vi "Trajectory_Controller.vi"(0 "Error In":errorcluster, 1 "reset":dbl, 2 "Interpolation activator":bool, 3 "Abort Trajectory":bool, 4 "Controller Data In":refnum<data-value>, 5 "Configuration":T1={"Accelerometer Bias"={"X (m/s)"=0.0, "Y (m/s)"=0.0, "Z (m/s)"=0.0}, "Gyroscope Bias"={"X (m/s)"=0.0, "Y (m/s)"=0.0, "Z (m/s)"=0.0}, "Steering Motor Gear Ratio"=611.0, "Steering Pully Gear Ratio"=1.0, "Steering Encoder CPR"=500.0, "Steering Motor Max RPM"=4000.0, "Wheelbase (m)"=1.12, "Fork Angle (rad)"=1.3, "Balancing Controller"={"Kp (/s)"=1.0, "Kd (1)"=1.0}, "Max Allowed Steering Angle (rad)"=0.7, "Task Periods"={"Emergency Stop (us)"=10000, "IMU (us)"=10000, "Steering Motor Encoder (us)"=10000, "State Estimator (us)"=10000, "Balancing Controller (us)"=10000, "GNSS (us)"=10000, "Logging (us)"=50000, "Drive Motor (us)"=100000, "Visualization (us)"=50000}, "Drive Motor Gear Ratio"=0.7, "lr"=0.0, "lf"=0.0, "lambda"=0.0, "k1"=0.0, "k2"=0.0, "e1_max"=0.0, "Ad_tmin"=0.0, "Bd_tmin"=0.0, "C_tmin"=0.0, "D_tmin"=0.0, "Wheel radius"=0.311, "Ad_tmax"=0.95971, "Bd_tmax"=0.01, "C_tmax"=2.20588, "D_tmax"=0.0, "Vmin"=2.20588, "Vmax"=0.0}, 7 "State Estimate In":refnum<data-value>, 8 "Constant V matrixmat":dbl, 9 "Reset and Init trajectory":bool, 11 "RefTraj in":refnum<data-value>, 12 "Trajectory In":refnum<data-value>, 13 "Measurement In":refnum<data-value>) -> (6 "Error out":errorcluster, 10 "Trajectory Out":refnum<data-value>, 14 "E1 limit":bool, 15 "E2 limit":bool)   [LabVIEW 2021]
uses:
  State Estimator/State Estimate.ctl
  Trajectory_Control.ctl
  Configuration/Configuration.ctl
  State Estimator/Measurements.ctl
  IMU/IMU Data.ctl
  Steering Motor Encoder/Steering Motor Encoder Data.ctl
  GNSS/GNSS Data.ctl
  Logging/Controller Data.ctl
  Drive Motor/Drive Motor Data.ctl
  Steering Motor/Steering Motor Data.ctl
panel:
  out "Numeric":dbl
  out "Controller Data Out":refnum<data-value>
  out "lat_con":dbl
  out "head con":dbl
  out "delta":dbl
  out "State Estimate Out":refnum<data-value>
  out "RefTraj out":refnum<data-value>
  out "Measurement Out":refnum<data-value>
  out "size(s)":i32[](array[numeric])
  out "error2":dbl
  out "error1":dbl
  out "Rollref":dbl
  out "Closestpoint":dbl
  in  "path in":path=path "libtrajectory_controller.so"
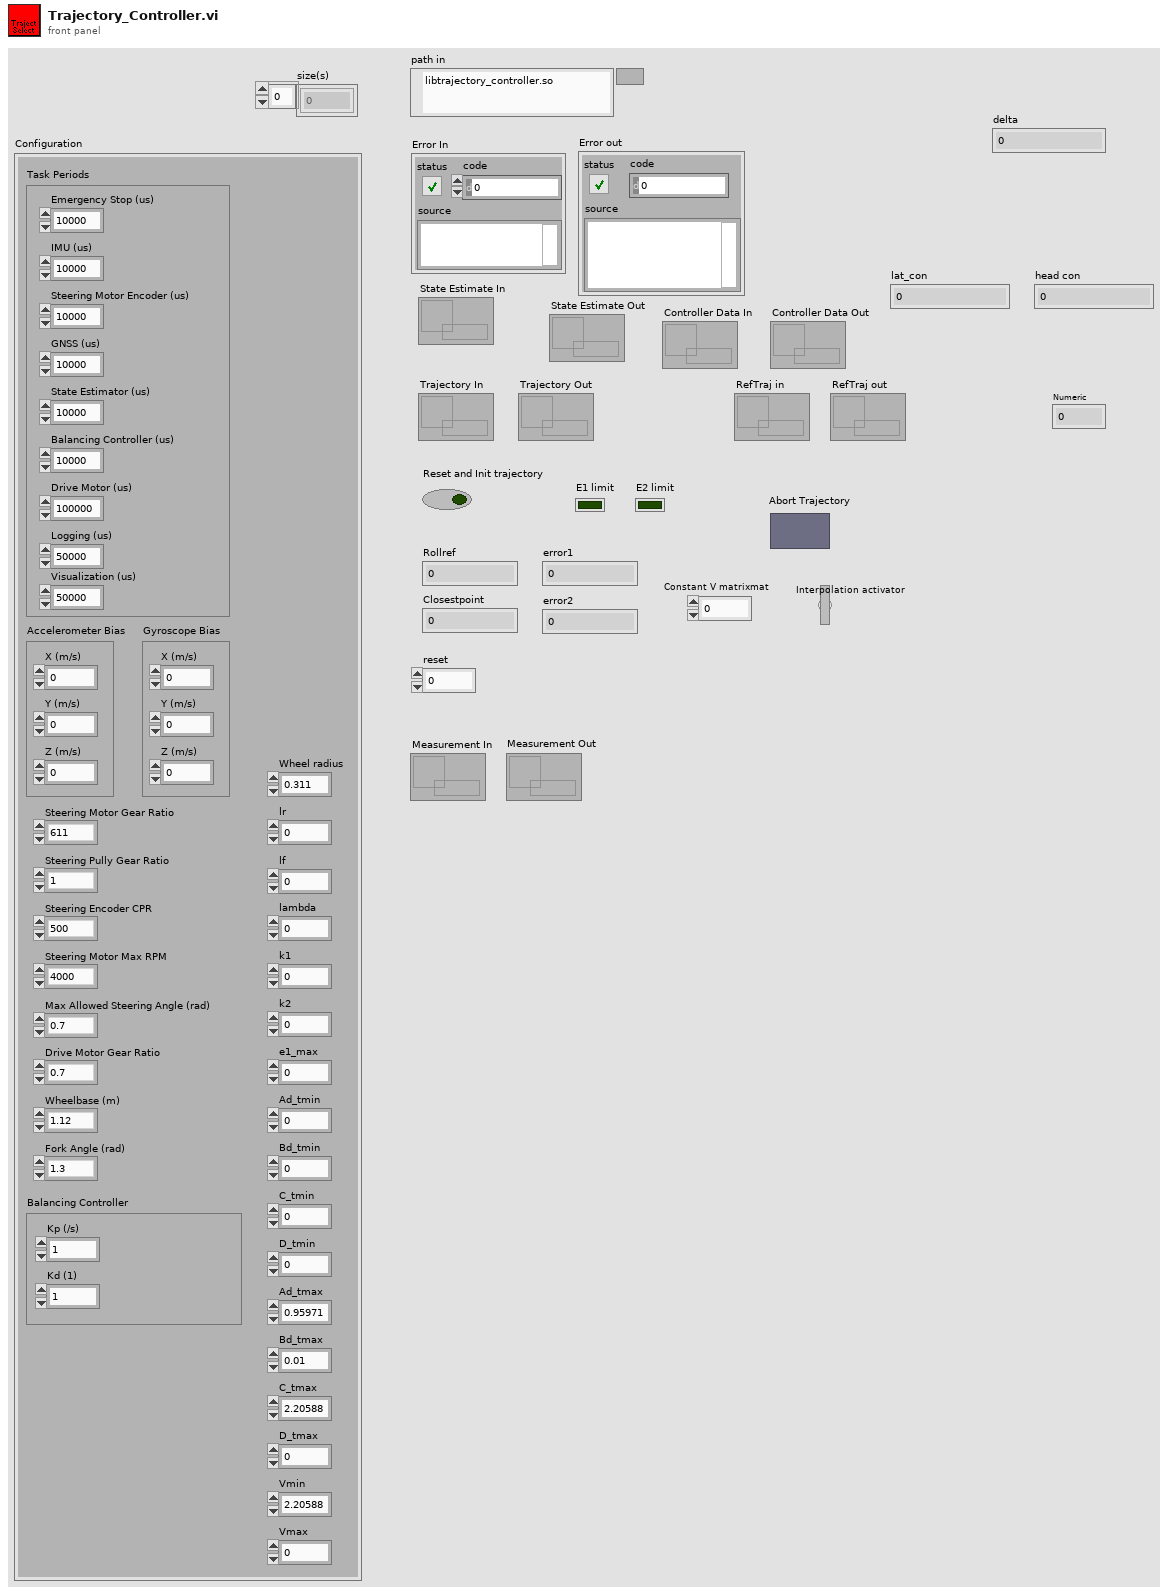
[diagram p1: front panel]
types:
  T1 = typedef "Configuration.ctl" = cluster{"Accelerometer Bias":cluster{"X (m/s)":dbl, "Y (m/s)":dbl, "Z (m/s)":dbl}, "Gyroscope Bias":cluster{"X (m/s)":dbl, "Y (m/s)":dbl, "Z (m/s)":dbl}, "Steering Motor Gear Ratio":dbl, "Steering Pully Gear Ratio":dbl, "Steering Encoder CPR":dbl, "Steering Motor Max RPM":dbl, "Wheelbase (m)":dbl, "Fork Angle (rad)":dbl, "Balancing Controller":cluster{"Kp (/s)":dbl, "Kd (1)":dbl}, "Max Allowed Steering Angle (rad)":dbl, "Task Periods":cluster{"Emergency Stop (us)":i64, "IMU (us)":i64, "Steering Motor Encoder (us)":i64, "State Estimator (us)":i64, "Balancing Controller (us)":i64, "GNSS (us)":i64, "Logging (us)":i64, "Drive Motor (us)":i64, "Visualization (us)":i64}, "Drive Motor Gear Ratio":dbl, "lr":dbl, "lf":dbl, "lambda":dbl, "k1":dbl, "k2":dbl, "e1_max":dbl, "Ad_tmin":dbl, "Bd_tmin":dbl, "C_tmin":dbl, "D_tmin":dbl, "Wheel radius":dbl, "Ad_tmax":dbl, "Bd_tmax":dbl, "C_tmax":dbl, "D_tmax":dbl, "Vmin":dbl, "Vmax":dbl}
  T2 = typedef "Trajectory_Control.ctl" = cluster{"Rollref":dbl, "Closestpoint":dbl, "Error1":dbl, "Error2":dbl, "Dpsiref_cont":dbl, "Lateral_cont":dbl, "Heading_cont":dbl, "Reset_traj":dbl, "Iteration":dbl, "E1 limit":u32, "E2 limit":u32, "Vref":dbl}
  T3 = typedef "Measurements.ctl" = cluster{"IMU Data":T4, "Steering Motor Encoder Data":T5, "GNSS Data":T6}
  T4 = typedef "IMU Data.ctl" = cluster{"Gyroscope":cluster{"X (rad/s)":dbl, "Y (rad/s)":dbl, "Z (rad/s)":dbl}, "Accelerometer":cluster{"X (m/s^2)":dbl, "Y (m/s^2)":dbl, "Z (m/s^2)":dbl}, "Flag IMU":dbl}
  T5 = typedef "Steering Motor Encoder Data.ctl" = cluster{"Encoder Position (counts)":i32, "Steering Angle (rad)":dbl, "Steering Encoder Iteration":dbl}
  T6 = typedef "GNSS Data.ctl" = cluster{"Latitude (rad)":dbl, "Longitude (rad)":dbl, "Altitude (m)":dbl, "Speed (m/s)":dbl, "Heading (rad)":dbl, "Fix Quality":i32, "Number of Satellites":i32, "Latitude (deg)":dbl, "Longitude (deg)":dbl, "Flag GNSS":dbl}
  T7 = typedef "Controller Data.ctl" = cluster{"Drive Motor Data":T8, "Steering Motor Data":T9}
  T8 = typedef "Drive Motor Data.ctl" = cluster{"Angular Speed (rad/s)":dbl, "Input Current (A)":dbl, "Motor Current (A)":dbl, "MOSFET Temperature (deg C)":dbl, "Reference Speed (rad/s)":dbl, "PI Current (A)":dbl, "Ki":dbl, "Kp":dbl}
  T9 = typedef "Steering Motor Data.ctl" = cluster{"PWM":dbl, "Steering Angle Rate (rad/s)":dbl, "input balancing":dbl}
  T10 = typedef "State Estimate.ctl" = cluster{"X (m)":dbl, "Y (m)":dbl, "Psi (rad)":dbl, "Roll (rad)":dbl, "Roll Rate (rad/s)":dbl, "delta":dbl, "velocity":dbl, "Iterations":dbl}
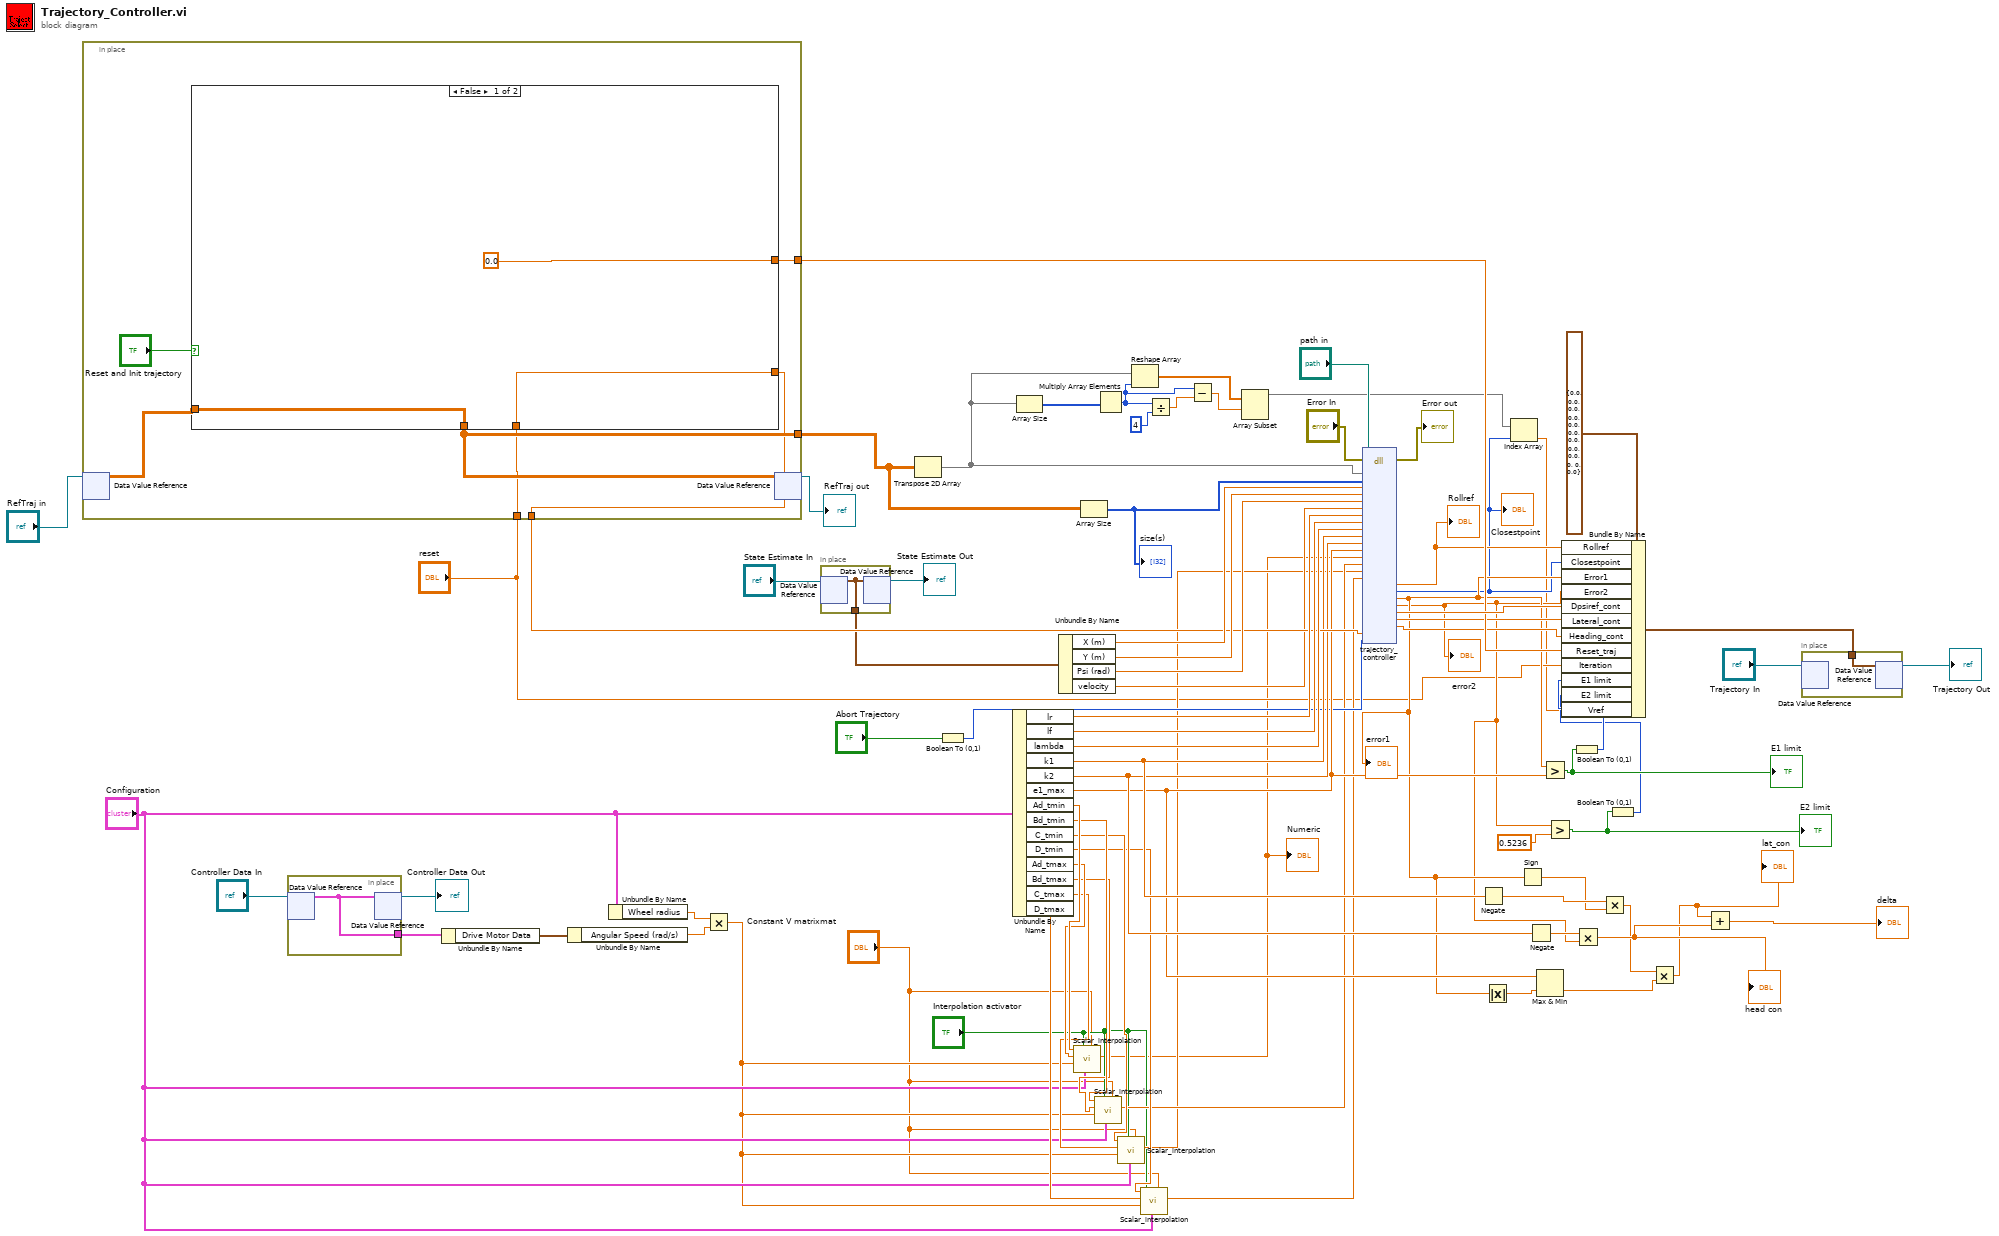
[diagram p0: block diagram]
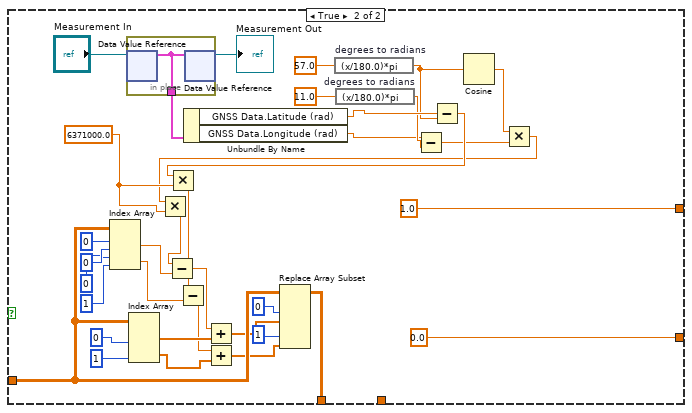
[diagram p2: hidden frame]
diagram:
  n1 = in-place {
    in-place-border: [w85] -> w63
    in-place-border: [w87] -> w13
    in-place-border: [w83] -> w65
    in-place-border: "reset" -> [w82]
    n2 = in-place-dvr #1("RefTraj in") -> (w86:dbl[][])  [unwired: 1 out]
    n3 = case shown="False" "Reset and Init trajectory" {
      tunnel: [w88 0.0] -> w85
      tunnel: [w90 w108] -> w87
      tunnel: w86 -> [w90 w118]
      tunnel: [0.0 1.0] -> w83
      tunnel: w82 -> [w88 _]
      frame False {
      }
      frame True {
        w120 = 6371000.0
        n4 = Index Array(array=w118, index (row) #1=0, index (col) #1=0, index (row) #2=0, index (col) #2=1) -> (element #1=w92:dbl, element #2=w113:dbl)
        n5 = in-place {
          in-place-border: [w127] -> w123
          n6 = in-place-dvr #2("Measurement In") -> (w127:T3)  [unwired: 1 out]
          n7 = in-place-dvr #2(w127) -> (→"Measurement Out":refnum<data-value>)  [unwired: 1 out]
        }
        n8 = Index Array(array=w118, index (col) #1=0, index (col) #2=1) -> (element #1=w121:dbl[], element #2=w110:dbl[])  [unwired: 2 in]
        n9 = Unbundle By Name(w123) -> ("GNSS Data.Latitude (rad)"=w102:dbl, "GNSS Data.Longitude (rad)"=w99:dbl)
        n10 = expression code="(x/180.0)*pi" "degrees to radians"(57.0 ("y")) -> (w97:dbl)
        n11 = expression code="(x/180.0)*pi" "degrees to radians"(11.0 ("y")) -> (w100:dbl)
        n12 = Subtract(x=w99, y=w100) -> (x-y=w95:dbl)
        n13 = Subtract(x=w102, y=w97) -> (x-y=w98:dbl)
        n14 = Multiply(x=w98, y=w120) -> (x*y=w119:dbl)
        n15 = Subtract(x=w119, y=w113) -> (x-y=w111:dbl)
        n16 = Add(x=w111, y=w110) -> (x+y=w109:dbl[])
        n17 = Cosine(x=w97) -> (cos(x)=w96:dbl)
        n18 = Multiply(x=w96, y=w95) -> (x*y=w94:dbl)
        n19 = Multiply(x=w94, y=w120) -> (x*y=w93:dbl)
        n20 = Subtract(x=w93, y=w92) -> (x-y=w122:dbl)
        n21 = Add(x=w122, y=w121) -> (x+y=w112:dbl[])
        n22 = Replace Array Subset(array=w118, new element #1=w112, index (col) #1=0, new element #2=w109, index (col) #2=1) -> (w108:dbl[][])  [unwired: 2 in]
      }
    }
    n23 = in-place-dvr #1(w87) -> (→"RefTraj out":refnum<data-value>)  [unwired: 1 out]
  }
  n24 = in-place {
    in-place-border: [w128] -> w21
    n25 = in-place-dvr #3("Controller Data In") -> (w128:T7)  [unwired: 1 out]
    n26 = in-place-dvr #3(w128) -> (→"Controller Data Out":refnum<data-value>)  [unwired: 1 out]
  }
  n27 = Unbundle By Name(w21) -> ("Drive Motor Data"=w20:T8)
  n28 = Unbundle By Name(w20) -> ("Angular Speed (rad/s)"=w17:dbl)
  n29 = Unbundle By Name("Configuration") -> ("Wheel radius"=w16:dbl)
  n30 = Multiply(x=w16, y=w17) -> (x*y=w15:dbl)
  n31 = in-place {
    in-place-border: [w129] -> w24
    n32 = in-place-dvr #4("State Estimate In") -> (w129:T10)  [unwired: 1 out]
    n33 = in-place-dvr #4(w129) -> (→"State Estimate Out":refnum<data-value>)  [unwired: 1 out]
  }
  n34 = Transpose 2D Array(2D array=w13) -> (transposed array=w5:dbl[][])
  n35 = Boolean To (0,1)(Boolean="Abort Trajectory") -> (0, 1=w36:i16)
  n36 = Unbundle By Name("Configuration") -> ("lr"=w72:dbl, "lf"=w71:dbl, "lambda"=w70:dbl, "k1"=w59:dbl, "k2"=w58:dbl, "e1_max"=w52:dbl, "Ad_tmin"=w35:dbl, "Bd_tmin"=w33:dbl, "C_tmin"=w31:dbl, "D_tmin"=w29:dbl, "Ad_tmax"=w34:dbl, "Bd_tmax"=w32:dbl, "C_tmax"=w30:dbl, "D_tmax"=w28:dbl)
  n37 = Array Size(array=w5) -> (size(s)=w14:i32[])
  n38 = Unbundle By Name(w24) -> ("X (m)"=w79:dbl, "Y (m)"=w78:dbl, "Psi (rad)"=w77:dbl, "velocity"=w60:dbl)
  n39 = call "Scalar_interpolation.vi"("Constant V for matrixmat"="Constant V matrixmat", "Configuration"="Configuration", "Interpolation activator"="Interpolation activator", "Vest"=w15, "Max"=w34, "Min"=w35) -> ("Final value"=w1:dbl)  [unwired: 5 in]
  "Numeric" <- w1
  n40 = Array Size(array=w13) -> (size(s)=w66:i32[])
  "size(s)" <- w66
  n41 = call "Scalar_interpolation.vi"("Constant V for matrixmat"="Constant V matrixmat", "Configuration"="Configuration", "Interpolation activator"="Interpolation activator", "Vest"=w15, "Max"=w32, "Min"=w33) -> ("Final value"=w27:dbl)  [unwired: 5 in]
  n42 = Multiply Array Elements(1:w14) -> (0:w8:i32)
  n43 = call "Scalar_interpolation.vi"("Constant V for matrixmat"="Constant V matrixmat", "Configuration"="Configuration", "Interpolation activator"="Interpolation activator", "Vest"=w15, "Max"=w30, "Min"=w31) -> ("Final value"=w26:dbl)  [unwired: 5 in]
  n44 = Reshape Array(w5, w8) -> (w6:dbl[])
  n45 = call "Scalar_interpolation.vi"("Constant V for matrixmat"="Constant V matrixmat", "Configuration"="Configuration", "Interpolation activator"="Interpolation activator", "Vest"=w15, "Max"=w28, "Min"=w29) -> ("Final value"=w25:dbl)  [unwired: 5 in]
  n46 = Divide(x=w8, y=4) -> (x/y=w11:dbl)
  n47 = Subtract(x=w8, y=w11) -> (x-y=w7:dbl)
  n48 = Array Subset(array=w6, index=w7) -> (w4:dbl[])  [unwired: 1 in]
  n49 = dll-call lib="libtrajectory_controller.so" fn="trajectory_controller"(path in="path in", error in="Error In", "Traj"=w5, "traj_size"=w66, "X"=w79, "Y"=w78, "Psi"=w77, "v"=w60, "lr"=w72, "lf"=w71, "lambda"=w70, "k1"=w59, "k2"=w58, "e1max"=w52, "Adt"=w1, "Bdt"=w27, "Ct"=w26, "Dt"=w25, "Reset"=w63, "abort"=w36) -> (error out=→"Error out":errorcluster, "Rollref"=w62:dbl, "Closestpoint"=w10:i32, "error1"=w45:dbl, "error2"=w44:dbl, "dpsiref_cont"=w69:dbl, "Lateral_cont"=w46:dbl, "Heading_cont"=w47:dbl)  [unwired: 27 in, 1 out]
  "Closestpoint" <- w10
  "Rollref" <- w62
  "error1" <- w45
  "error2" <- w44
  n50 = Negate(x=w59) -> (-x=w57:dbl)
  n51 = Absolute Value(x=w45) -> (abs(x)=w51:dbl)
  n52 = Index Array(array=w4, index=w10) -> (element=w9:dbl)
  n53 = Sign(1:w45) -> (0:w53:dbl)
  n54 = Negate(x=w58) -> (-x=w56:dbl)
  n55 = Max & Min(x=w52, y=w51) -> (min(x,y)=w50:dbl)  [unwired: 1 out]
  n56 = Greater?(x=w45, y=w52) -> (0:w40:bool)
  "E1 limit" <- w40
  n57 = Greater?(x=w44, y=0.5236) -> (0:w41:bool)
  "E2 limit" <- w41
  n58 = Boolean To (0,1)(Boolean=w40) -> (0, 1=w39:i16)
  n59 = Multiply(x=w56, y=w44) -> (x*y=w55:dbl)
  "head con" <- w55
  n60 = Multiply(x=w57, y=w53) -> (x*y=w49:dbl)
  n61 = Boolean To (0,1)(Boolean=w41) -> (0, 1=w38:i16)
  n62 = Bundle By Name(cluster=T2 {"Rollref"=0.0, "Closestpoint"=0.0, "Error1"=0.0, "Error2"=0.0, "Dpsiref_cont"=0.0, "Lateral_cont"=0.0, "Heading_cont"=0.0, "Reset_traj"=0.0, "Iteration"=0.0, "E1 limit"=0, "E2 limit"=0, "Vref"=0.0} ("Trajectory (Debug)"), "Rollref"=w62, "Closestpoint"=w10, "Error1"=w45, "Error2"=w44, "Dpsiref_cont"=w69, "Lateral_cont"=w46, "Heading_cont"=w47, "Reset_traj"=w65, "Iteration"="reset", "E1 limit"=w39, "E2 limit"=w38, "Vref"=w9) -> (w42:T2)
  n63 = Multiply(x=w49, y=w50) -> (x*y=w48:dbl)
  "lat_con" <- w48
  n64 = Add(x=w48, y=w55) -> (x+y=→"delta":dbl)
  n65 = in-place {
    in-place-border: w42 -> [w130]
    n66 = in-place-dvr #5("Trajectory In") -> ()  [unwired: 2 out]
    n67 = in-place-dvr #5(w130) -> (→"Trajectory Out":refnum<data-value>)  [unwired: 1 out]
  }
